vi "DropIn Get Button Clicks - Stub.vi"(5 "file (use dialog)":path=path "C:/Solutions/LabVIEW Advanced Architectures/Test Drop In.txt", 11 "error in (no error)":errorcluster) -> (15 "error out":errorcluster)   [LabVIEW 2011]
doc: "This is the starting point for the drop ins exercise. Given a path, the drop in will record all button value change events and document the time, relative to a zero time when the parent is initially run, at which the button press occured.\n\nAAL 9/09"
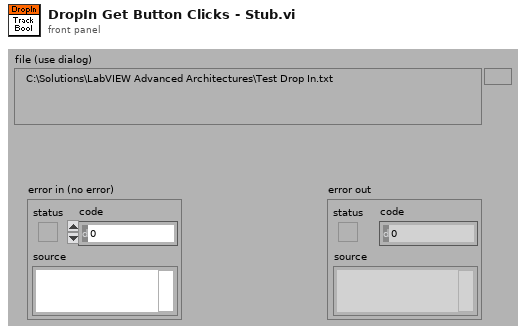
[diagram p1: front panel]
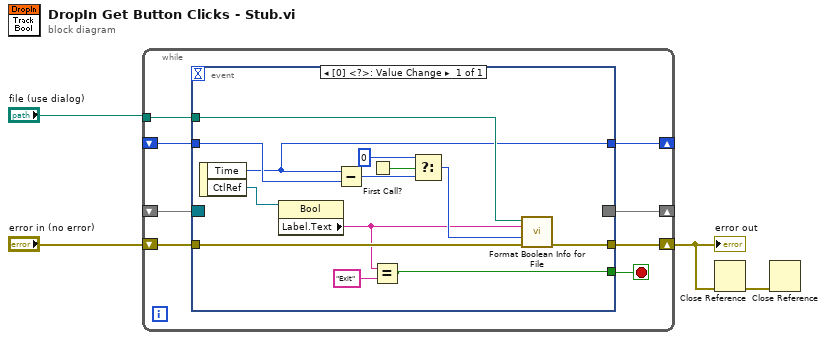
[diagram p0: block diagram]
diagram:
  n1 = while {
    shift-right: [w9] -> _
    shift-left: _ -> [w12]
    shift-right: [w10] -> w3
    shift-left: "error in (no error)" -> [w11]
    tunnel: "file (use dialog)" -> [w8]
    shift-right: [w6] -> _
    shift-left: _ -> [w7]
    stop <- w5 stop-if-true
    n2 = event shown="[0] <?>: Value Change" {
      selector: w12 -> [_]
      dyn-events: [_] -> w9
      timeout: _ -> [_]
      tunnel: w11 -> [w24]
      tunnel: [w23] -> w10
      tunnel: w8 -> [w22]
      tunnel: w7 -> [w25]
      tunnel: [w21] -> w6
      tunnel: [w13] -> w5
      event Value Change {
        n3 = event-data() -> ("Time"=w21:u32, "CtlRef"=w16:refnum<vi>)  [unwired: 1 out]
        n4 = property class="Bool"(reference=w16) -> ("Label.Text"=w15:string)  [unwired: 1 in, 2 out]
        n5 = Subtract(x=w21, y=w25) -> (x-y=w19:u32)
        n6 = First Call?() -> (First Call?: T/F=w20:bool)
        n7 = Equal?(x=w15, y="Exit") -> (x = y?=w13:bool)
        n8 = Select(t=u32 0, s=w20, f=w19) -> (s? t:f=w18:u32)
        n9 = call "Format Boolean Info for File.vi"("File Name"=w22, "Label Name"=w15, "Time (msec)"=w18, "error in (no error)"=w24) -> ("error out"=w23:errorcluster)  [unwired: 1 in, 5 out]
      }
    }
  }
  "error out" <- w3
  n10 = Close Reference(error in (no error)=w3) -> (error out=w2:errorcluster)  [unwired: 1 in]
  n11 = Close Reference(error in (no error)=w2) -> ()  [unwired: 1 in, 1 out]
